vi "Send Iteration Message.vi"(8 "error in (no error)":errorcluster, 10 "Iteration Msg":refnum<class "Message.lvclass">, 11 "Iterator NR Actor in":refnum<class "Iterator NR Actor.lvclass">) -> (0 "error out":errorcluster)   [LabVIEW 2023, in "Iterator Actor.lvlib" / "Iterator NR Actor.lvclass"]
uses:
  Iterator NR Actor.lvclass
  <vilib>/ActorFramework/Message Enqueuer/Message Enqueuer.lvclass
  <vilib>/ActorFramework/Actor/Actor.lvclass
  Iterator NR Actor Messages/Abstract Iteration Msg/Abstract Iteration Msg.lvclass
  <userlib>/_OpenG.lib/lvdata/lvdata.llb/openg_variant.lvlib
  <vilib>/ActorFramework/Batch Msg/Batch Msg.lvclass
  <vilib>/ActorFramework/Message/Message.lvclass
  Iterator NR Actor Messages/Request Iteration Notification Msg/Request Iteration Notification Msg.lvclass
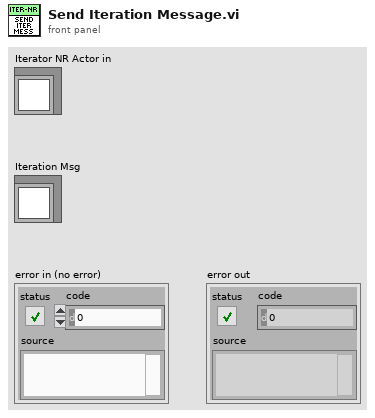
[diagram p1: front panel]
types:
  T1 = typedef "Iterator Actor.lvlib/Abstract Iterator Actor.lvclass/Iterator Settings.ctl" = cluster{"Prepare timeout (ms)":i32, "Iterate timeout (ms)":i32, "Conclude timeout (ms)":i32, "Iterate period (ms)":i32, "Number of iterations":i32, "Time before stop (ms)":i32, "Active Stop Conditions":T2, "Prepare Msg":refnum<class "Message.lvclass">, "Iterate Msg":refnum<class "Message.lvclass">, "Conclude Msg":refnum<class "Message.lvclass">, "Iterations End Report":refnum<class "Iterator Report Iterations End Msg.lvclass">, "Message Priority (Normal)":T3}
  T2 = typedef "Iterator Actor.lvlib/Abstract Iterator Actor.lvclass/Active Stop Conditions.ctl" = cluster{"Number of Iterations":bool, "Time Elapsed":bool, "Iteration Result":bool}
  T3 = typedef "Actor Framework.lvlib/Message Enqueuer.lvclass/Message Priority.ctl" = enum16{"Low", "Normal", "High"}
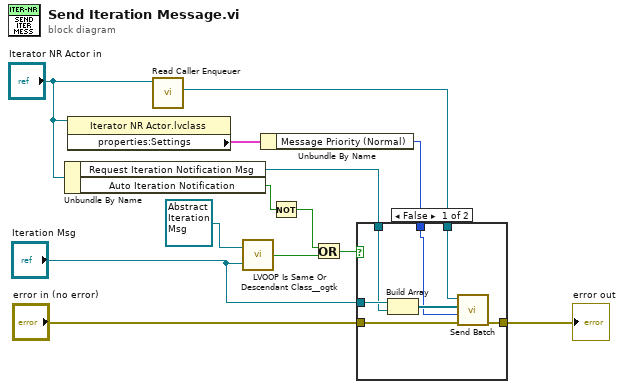
[diagram p0: block diagram]
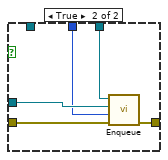
[diagram p2: hidden frame]
diagram:
  n1 = Unbundle By Name("Iterator NR Actor in") -> ("Request Iteration Notification Msg"=w4:refnum<class "Request Iteration Notification Msg.lvclass">, "Auto Iteration Notification"=w6:bool)
  n2 = property class="Iterator NR Actor.lvclass"(reference="Iterator NR Actor in") -> ("properties:Settings"=w2:T1)  [unwired: 1 in, 2 out]
  n3 = call <vilib>:"Read Caller Enqueuer.vi"("Actor"="Iterator NR Actor in") -> ("Caller Enqueuer"=w13:refnum<class "Message Enqueuer.lvclass">)  [unwired: 10 in]
  n4 = call <userlib>:"LVOOP Is Same Or Descendant Class__ogtk.vi"("Possible Descendant Object"="Iteration Msg", "Object"=refnum<class "Abstract Iteration Msg.lvclass"> refnum ("Iterator Actor.lvlib:Abstract Iteration Msg.lvclass")) -> ("Is Same Class or Descendant?"=w8:bool)
  n5 = Unbundle By Name(w2) -> ("Message Priority (Normal)"=w1:T3)
  n6 = Not(x=w6) -> (.not. x?=w5:bool)
  n7 = Or(x=w5, y=w8) -> (x .or. y?=w7:bool)
  n8 = case shown="False" w7 {
    tunnel: w13 -> [w15 w25]
    tunnel: [w19 w24] -> w12
    tunnel: "error in (no error)" -> [w20 w23]
    tunnel: "Iteration Msg" -> [w18 w22]
    tunnel: w4 -> [w17 _]
    tunnel: w1 -> [w14 w21]
    frame False {
      n9 = Build Array(w18, w17) -> (w16:refnum<class "Message.lvclass">[])
      n10 = call <vilib>:"Send Batch.vi"("error in (no error)"=w20, "Message Priority (Normal)"=w14, "Messages Array"=w16, "Message Enqueuer"=w15) -> ("error out"=w19:errorcluster)  [unwired: 7 in]
    }
    frame True {
      n11 = call <vilib>:"Enqueue.vi"("error in (no error)"=w23, "Message Priority (Normal)"=w21, "Message"=w22, "Message Enqueuer in"=w25) -> ("error out"=w24:errorcluster)  [unwired: 6 in, 1 out]
    }
  }
  "error out" <- w12
